vi "Production_count_sum.vi"(8 "PROD_COUNT":string[](array[string]), 9 "Table 3":string[][](array[string]), 10 "date count":string[](array[string]), 11 "Founded dates":string[](array[string])) -> (2 "sum":i32[](array[numeric]), 3 "Array 3":string[][](array[string]))   [LabVIEW 2017]
panel:
  out "Array":string[](array[string])
  out "Array 2":i32[](array[numeric])
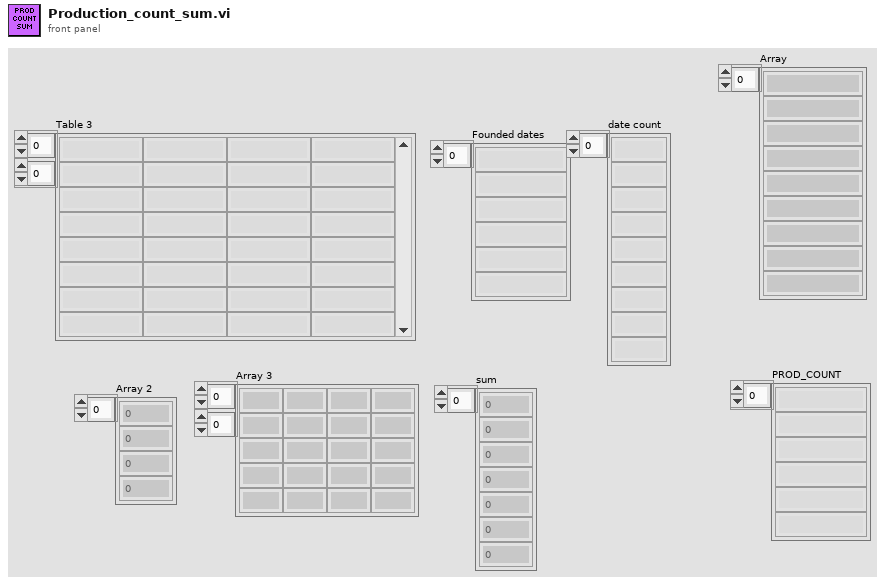
[diagram p1: front panel]
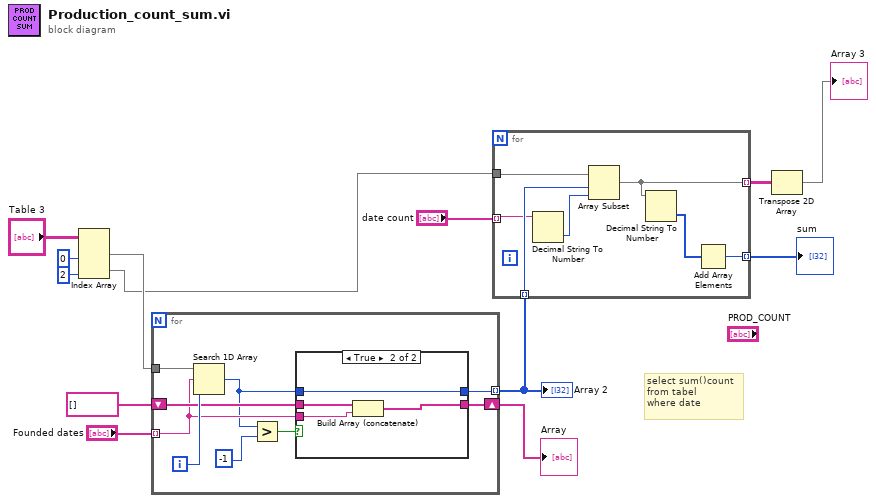
[diagram p0: block diagram]
diagram:
  # "select sum()count\nfrom tabel\nwhere date"
  n1 = Index Array(array="Table 3", index (col) #1=0 ("disabled index (col)"), index (col) #2=2 ("index (col)")) -> (element #1=w9:string[], element #2=w6:string[])  [unwired: 2 in]
  n2 = for {
    tunnel: "Founded dates" -> [w17] mode=indexing
    shift-right: [w19] -> w1
    shift-left: string[] [] -> [w18]
    tunnel: w9 -> [w16]
    tunnel: [w15] -> w8 mode=indexing
    i -> [w22]
    n3 = Search 1D Array(1D array=w16, element=w17, start index (0)=w22) -> (index of element=w14:i32)
    n4 = Greater?(x=w14, y=-1) -> (0:w20:bool)
    n5 = case shown="True" w20 {
      tunnel: w18 -> [w24 w28]
      tunnel: [w24 w27] -> w19
      tunnel: w17 -> [_ w26]
      tunnel: [w23 w25] -> w15
      tunnel: w14 -> [w23 w25]
      frame False {
      }
      frame True {
        n6 = Build Array (concatenate)(w28, w26) -> (w27:string[])
      }
    }
  }
  "Array 2" <- w8
  "Array" <- w1
  n7 = for {
    tunnel: w6 -> [w35]
    tunnel: w8 -> [w34] mode=indexing
    tunnel: "date count" -> [w33] mode=indexing
    tunnel: [w31] -> w7 mode=indexing
    tunnel: [w29] -> w3 mode=indexing
    n8 = Decimal String To Number(string=w33) -> (number=w32:i32)  [unwired: 2 in, 1 out]
    n9 = Array Subset(array=w35, index=w34, length=w32) -> (w31:string[])
    n10 = Decimal String To Number(string=w31) -> (number=w30:i32[])  [unwired: 2 in, 1 out]
    n11 = Add Array Elements(numeric array=w30) -> (sum=w29:i32)
  }
  "sum" <- w3
  n12 = Transpose 2D Array(2D array=w7) -> (transposed array=→"Array 3":string[][])
